vi "Dummy_Func_VAR_dblX.vi"(10 "X":dbl, 11 "Variant":variant) -> (0 "Error":bool, 3 "NewX":dbl)   [LabVIEW 2019]
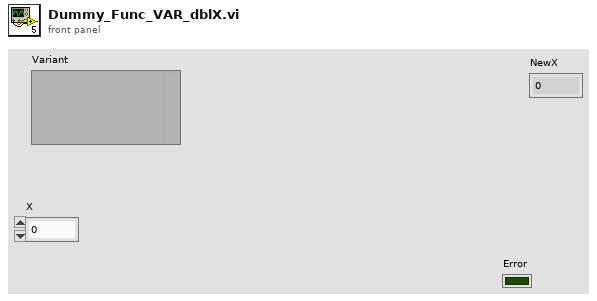
[diagram p1: front panel]
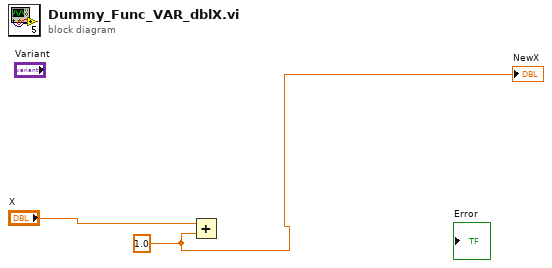
[diagram p0: block diagram]
diagram:
  w1 = 1.0 ("X")
  n1 = Add(x="X", y=w1) -> ()  [unwired: 1 out]
  "NewX" <- w1
